vi "Configure Trend Plot.vi"(6 "Trend Plot Type (0: Frequency)":i32(ring) items=["None", "Phase", "DelayRR", "DelayRF", "DelayFR", "DelayFF", "Frequency", "Mean", "Period", "Positive Duty", "Negative Duty", "Peak to Peak", "Cycle RMS", "Minimum", "Maximum", "Rise Time", "Fall Time", "Positive Width", "Negative Width", "Amplitude", "Cycle Mean", "High", "Low", "Positive Overshoot", "Negative Overshoot", "Cursor Mean", "Burst Width", "Positive Pulse Count", "Negative Pulse Count", "Rising Edge Count", "Falling Edge Count", "Area", "Cycle Area", "RMS", "Cursor RMS"], 7 "Trend Plot Source (0: Channel 1)":i32(ring) items=["Channel 1", "Channel 2", "Math", "Channel 1 - Channel 2", "Channel 2 - Channel 1", "Channel 1 - Math", "Math - Channel 1", "Channel 2-Math", "Math - Channel 2"], 8 "error in (no error)":errorcluster, 9 "Trend Plot State (0: Run)":i32(ring) items=["Run", "Stop"], 10 "Channel Number (1: Trend Plot 1)":i32(ring)=1 items=["Trend Plot 1"=1, "Trend Plot 2"=2], 11 "VISA resource name":refnum<visa-resource-name>) -> (0 "error out":errorcluster, 3 "VISA resource name out":refnum<visa-resource-name>)   [LabVIEW 2017, in "Tektronix TDS 200 1000 2000 Series.lvlib"]
doc: "Configures trend plot running state, source and type.\n\n<b>Note(s):</b>\nThis VI is only applicable for TBS1000B series models."
uses:
  Tektronix TDS 200 1000 2000 Series.lvlib
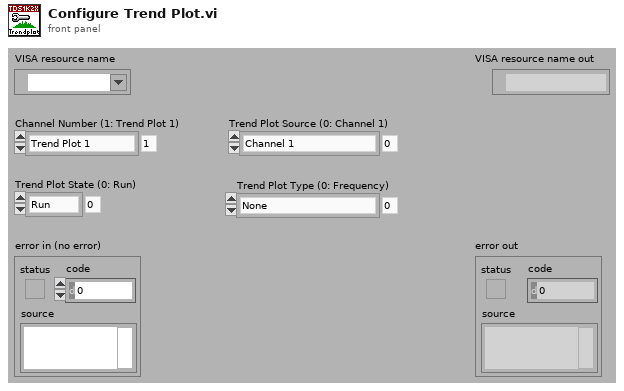
[diagram p1: front panel]
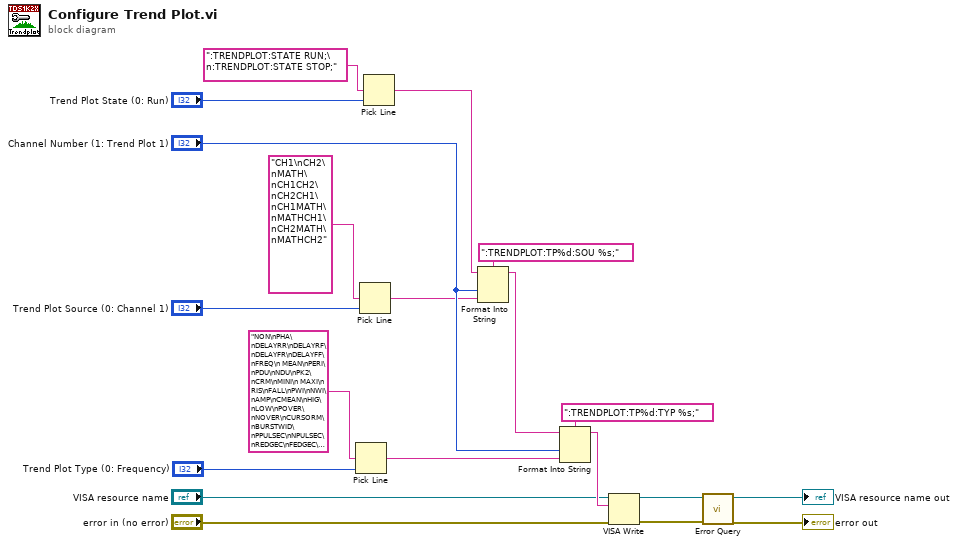
[diagram p0: block diagram]
diagram:
  n1 = Pick Line(multi-line string="NON\nPHA\nDELAYRR\nDELAYRF\nDELAYFR\nDELAYFF\nFREQ\n MEAN\nPERI\nPDU\nNDU\nPK2\nCRM\nMINI\n MAXI\n RIS\nFALL\nPWI\nNWI\nAMP\nCMEAN\nHIG\nLOW\nPOVER\nNOVER\nCURSORM\nBURSTWID\nPPULSEC\nNPULSEC\nREDGEC\nFEDGEC\nAREA\nCAREA\nRMS\nCURSORR", line index="Trend Plot Type (0: Frequency)") -> (output string=w12:string)  [unwired: 1 out]
  n2 = Pick Line(multi-line string="CH1\nCH2\nMATH\nCH1CH2\nCH2CH1\nCH1MATH\nMATHCH1\nCH2MATH\nMATHCH2", line index="Trend Plot Source (0: Channel 1)") -> (output string=w14:string)  [unwired: 1 out]
  n3 = Pick Line(multi-line string=":TRENDPLOT:STATE RUN;\n:TRENDPLOT:STATE STOP;", line index="Trend Plot State (0: Run)") -> (output string=w1:string)  [unwired: 1 out]
  n4 = Format Into String(format string=":TRENDPLOT:TP%d:SOU %s;", initial string=w1, "Channel Number (1: Trend Plot 1)", w14) -> (resulting string=w2:string)  [unwired: 1 in, 1 out]
  n5 = Format Into String(format string=":TRENDPLOT:TP%d:TYP %s;", initial string=w2, "Channel Number (1: Trend Plot 1)", w12) -> (resulting string=w5:string)  [unwired: 1 in, 1 out]
  n6 = VISA Write(VISA resource name="VISA resource name", write buffer=w5, error in (no error)="error in (no error)") -> (VISA resource name out=w11:refnum<visa-resource-name>, error out=w10:errorcluster)  [unwired: 1 out]
  n7 = call "Error Query.vi"("error in (no error)"=w10, "VISA resource name"=w11) -> ("error out"=→"error out":errorcluster, "VISA resource name out"=→"VISA resource name out":refnum<visa-resource-name>)  [unwired: 8 out]
